vi "ShortestAngle-Ether.vi"(9 "Current":dbl, 11 "Target":dbl) -> (3 "Shortest Correction":dbl)   [LabVIEW 2016]
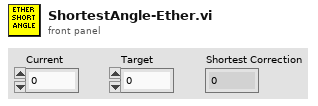
[diagram p1: front panel]
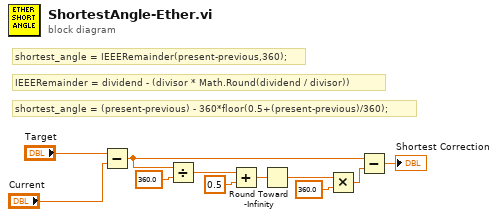
[diagram p0: block diagram]
diagram:
  # "shortest_angle = (present-previous) - 360*floor(0.5+(present-previous)/360);"
  # "shortest_angle = IEEERemainder(present-previous,360);"
  # "IEEERemainder = dividend - (divisor * Math.Round(dividend / divisor))"
  n1 = Subtract(x="Target", y="Current") -> (x-y=w5:dbl)
  n2 = Divide(x=w5, y=360.0) -> (x/y=w8:dbl)
  n3 = Add(x=w8, y=0.5) -> (x+y=w3:dbl)
  n4 = Round Toward -Infinity(1:w3) -> (0:w2:dbl)
  n5 = Multiply(x=w2, y=360.0) -> (x*y=w4:dbl)
  n6 = Subtract(x=w5, y=w4) -> (x-y=→"Shortest Correction":dbl)
